vi "Read PDF Details.vi"(0 "PDF Report Class in":refnum<class "PDF Report Class.lvclass">, 11 "error in (no error)":errorcluster) -> (4 "PDF Report Class out":refnum<class "PDF Report Class.lvclass">, 8 "PDF Details":T1, 15 "error out":errorcluster)   [LabVIEW 2019, in "PDF Report Class.lvclass"]
uses:
  <userlib>/Exaprom PDF/LV Class/PDF Report Class/PDF Report Class.lvclass
  <userlib>/Exaprom PDF/Controls/Initialization Controls/PDF Details.ctl
  <userlib>/Exaprom PDF/LV Class/PDF Report Class/PDF Report Class.lvclass/PDF Report Class.ctl
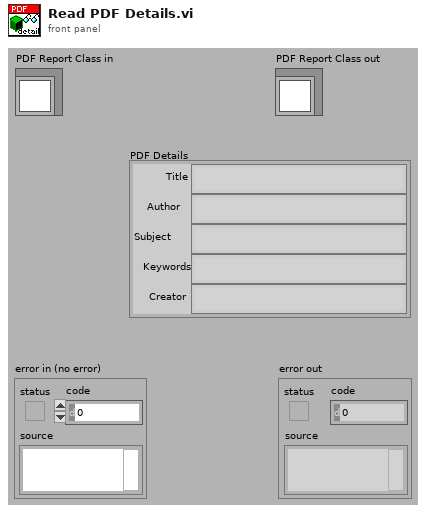
[diagram p1: front panel]
types:
  T1 = typedef "PDF Details.ctl" = cluster{"Title":string, "Author":string, "Subject":string, "Keywords":string, "Creator":string}
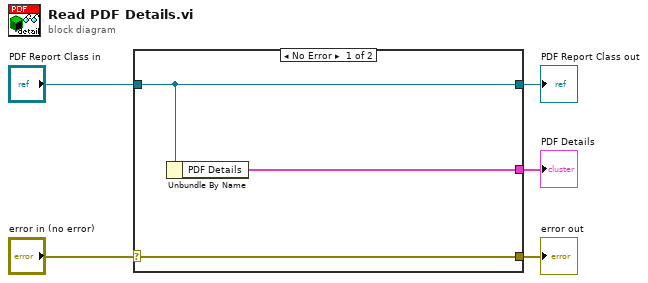
[diagram p0: block diagram]
diagram:
  n1 = case shown="No Error" "error in (no error)" {
    selector: "error in (no error)" -> [w8 w9]
    tunnel: [w8 w9] -> w4
    tunnel: [w7 w10] -> w2
    tunnel: "PDF Report Class in" -> [w7 w10]
    tunnel: [w6 _] -> w1
    frame No Error {
      n2 = Unbundle By Name(w7) -> ("PDF Details"=w6:T1)
    }
    frame Error {
    }
  }
  "error out" <- w4
  "PDF Report Class out" <- w2
  "PDF Details" <- w1
